vi "Gray's GUI.vi"() -> ()   [LabVIEW 2009]
uses:
  <vilib>/userDefined/High Color/nirio_resource_hc.ctl
  <vilib>/rvi/interface/nirviOpenFPGA/nirviOpenFPGA.xnode
  Brian Brain.lvproj_FPGA Target 2_Gray's Mod Motor C~4B.lvbitx
  <vilib>/FPGAPlugInAG/sbRIO-9642/nirviIntfOpen_sbRIO-9642.vi
  <vilib>/rvi/interface/nirviReadWriteControl/nirviReadWriteControl.xnode
  <vilib>/Utility/error.llb/Error Cluster From Error Code.vi
  <vilib>/rvi/errors/niLvFpgaAdjustHostInterfaceError.vi
  <vilib>/rvi/interface/common/niFpgaNodeNameForErrorReporting.ctl
  <vilib>/rvi/errors/niLvFpgaWhatHappensToTopLevelVI.ctl
  NiRioSrv.dll
panel:
  in  "resource name":T1="RIO0"
  in  "Steering Encoder Reset \nPosition Whole Rotations":i32
  in  "Drive Encoder Reset \nPosition Fractional":i32
  in  "Counts per Drive Position":i32=205386
  in  "Stop":bool=TRUE
  out "Drive Motor Speed (cpt)":fxp<+/-,20,1>
  out "Drive Encoder Delta (ticks)":u32
  in  "Drive Motor Speed Setpoint (mph)":fxp<+/-,20,7>
  in  "Drive Speed Proportional Control Feedback Gain":fxp<+/-,20,5>
  out "Drive Motor Speed (Volts)":fxp<+/-,20,5> format="%.17g"
  in  "Drive Conversion: \nmph to counts per tick":fxp<+/-,20,0>
  in  "Drive Encoder Offset":fxp<+/-,20,1>
  in  "Steering Proportional Control Feedback Gain":i32
  in  "Steer Motor Setpoint (degrees)":i8
  in  "Steering Encoder Offset from 0 counts":i32
  in  "Steering Conversion: degrees to ticks":i32
  out "Steering Motor Speed (Volts)":fxp<+/-,20,5> format="%.17g"
  out "Steering Position":i32
  out "Steering Encoder Index":i32
  out "Steering Encoder Raw":i32
  in  "Steering Encoder Reset":bool
  in  "Steering Encoder Reset \nPositions Fractional":i32
  out "Steering clock ticks/encoder count":u32
  in  "Drive Encoder Reset":bool
  in  "Drive Encoder Reset \nPosition Whole Rotations":i32
  out "Drive Encoder Index":i32
  out "Drive Position":i32
  # "Drive Motor Control"
  # "Steering Motor Control"
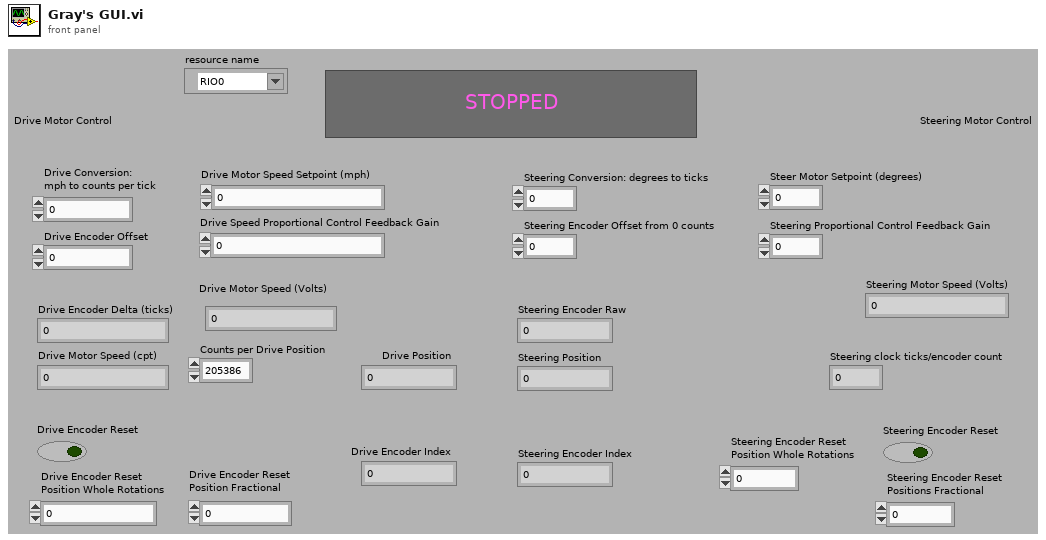
[diagram p1: front panel]
types:
  T1 = typedef "nirio_resource_hc.ctl" = tag
  T2 = typedef "niFpgaNodeNameForErrorReporting.ctl" = enum16{"Open FPGA VI Reference", "Read/Write Control", "Invoke Method: Abort", "Invoke Method: Acknowledge IRQ", "Invoke Method: Download", "Invoke Method: FIFO.Configure", "Invoke Method: FIFO.Read", "Invoke Method: FIFO.Start", "Invoke Method: FIFO.Stop", "Invoke Method: FIFO.Write", "Invoke Method: Reset", "Invoke Method: Run", "Invoke Method: Wait on IRQ", "Close FPGA VI Reference"}
  T3 = typedef "niLvFpgaWhatHappensToTopLevelVI.ctl" = enum16{"top level VI scripted behind XNode", "top level VI inlined behind XNode"}
  T4 = cluster{"signature":u8[], "vi signatures match":bool, "signature register address":u32, "reset register address":u32, "control register address":u32, "interrupt base address":u32, "Bitstream Version":u32, "DMA Configuration":cluster{"Name":string, "Depth":u32, "Write? (Deprecated:Use Implementation)":bool, "Physical Channel":u32, "Base Address":u32, "Data Width":u32, "Data Type":enum32{"Boolean", "I8", "I16", "I32", "I64", "U8", "U16", "U32", "U64", "FXP"}, "FXP Properties":variant, "Write Window Address":u32, "Implementation":enum16{"niFpgaTargetToHost", "niFpgaHostToTarget", "niFpgaPeerToPeerWriter", "niFpgaPeerToPeerReader", "niCoreTargetToHost", "niCoreHostToTarget"}, "Control Set":u32}[], "run when loaded?":bool, "reset register size in bits":u32, "compilation results xml":string}
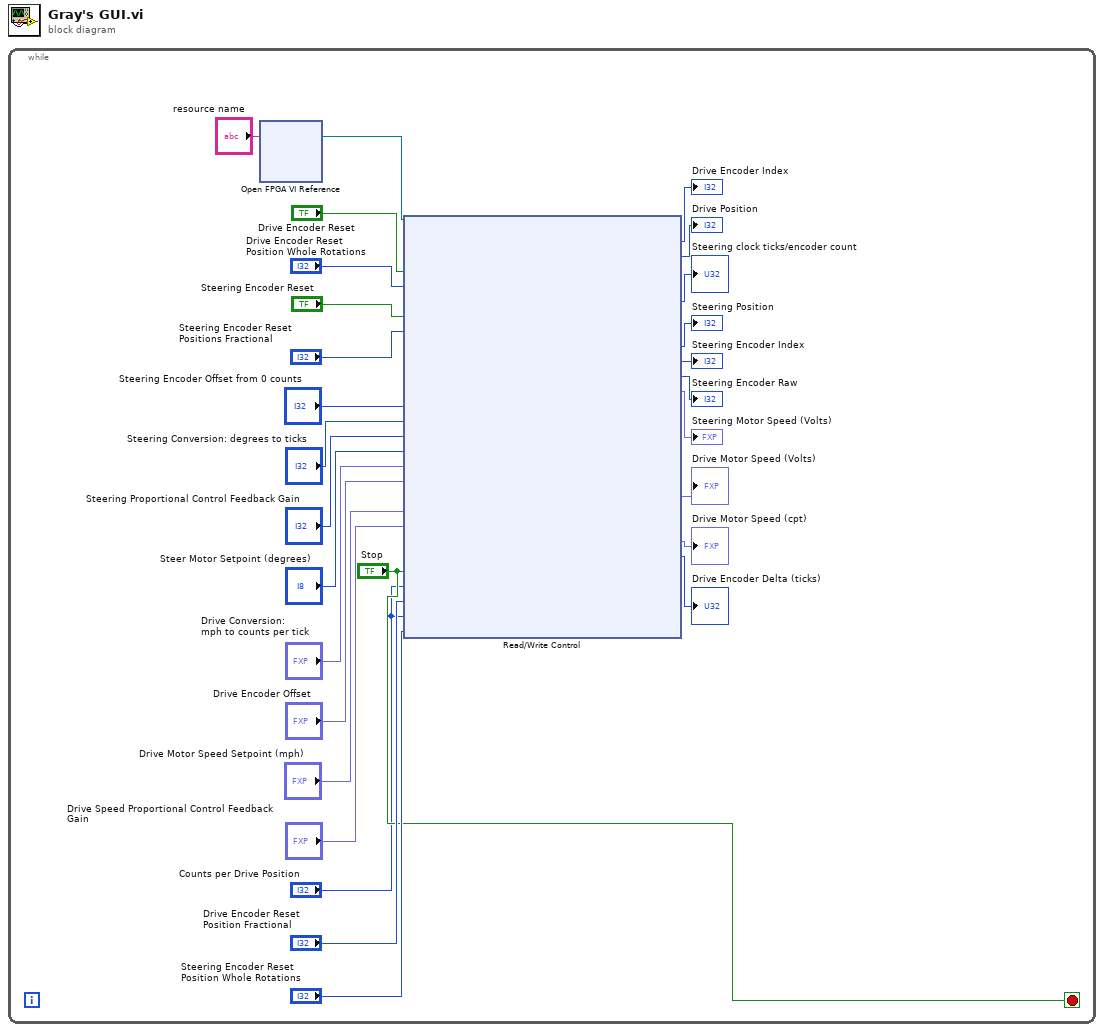
[diagram p0: block diagram]
diagram:
  n1 = while {
    stop <- "Stop" stop-if-true
    n2 = xnode "Open FPGA VI Reference"("resource name"="resource name") -> ("FPGA VI Reference Out"=w28:refnum<k20>)  [unwired: 1 in, 1 out]
    n3 = xnode "Read/Write Control"("FPGA VI Reference In"=w28, "Drive Encoder Reset"="Drive Encoder Reset", "Drive Encoder Reset  Position Whole Rotations"="Drive Encoder Reset \nPosition Whole Rotations", "Steering Encoder Reset"="Steering Encoder Reset", "Steering Encoder Reset  Positions Fractional"="Steering Encoder Reset \nPositions Fractional", "Steering Encoder Offset from 0 counts"="Steering Encoder Offset from 0 counts", "Steering Conversion: degrees to ticks"="Steering Conversion: degrees to ticks", "Steering Proportional Control Feedback Gain"="Steering Proportional Control Feedback Gain", "Steer Motor Setpoint (degrees)"="Steer Motor Setpoint (degrees)", "Drive Conversion:  mph to counts per tick"="Drive Conversion: \nmph to counts per tick", "Drive Encoder Offset"="Drive Encoder Offset", "Drive Motor Speed Setpoint (mph)"="Drive Motor Speed Setpoint (mph)", "Drive Speed Proportional Control Feedback Gain"="Drive Speed Proportional Control Feedback Gain", "Stop"="Stop", "Counts per Drive Position"="Counts per Drive Position", "Drive Encoder Reset  Position Fractional"="Drive Encoder Reset \nPosition Fractional", "Counts per Drive Position 2"="Counts per Drive Position", "Steering Encoder Reset  Position Whole Rotations"="Steering Encoder Reset \nPosition Whole Rotations") -> ("Drive Encoder Index"=→"Drive Encoder Index":i32, "Drive Position"=→"Drive Position":i32, "Steering clock ticks/encoder count"=→"Steering clock ticks/encoder count":u32, "Steering Position"=→"Steering Position":i32, "Steering Encoder Index"=→"Steering Encoder Index":i32, "Steering Encoder Raw"=→"Steering Encoder Raw":i32, "Steering Motor Speed (Volts)"=→"Steering Motor Speed (Volts)":fxp<+/-,20,5>, "Drive Motor Speed (Volts)"=→"Drive Motor Speed (Volts)":fxp<+/-,20,5>, "Drive Motor Speed (cpt)"=→"Drive Motor Speed (cpt)":fxp<+/-,20,1>, "Drive Encoder Delta (ticks)"=→"Drive Encoder Delta (ticks)":u32)  [unwired: 1 in, 2 out]
  }
